vi "Boolean_To_String.vi"(4 "boolean":bool) -> (1 "string":string)   [LabVIEW 2016, in "PyLVi.lvlib" / "PyLVi.lvclass"]
uses:
  PyLVi.lvclass
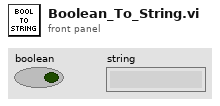
[diagram p1: front panel]
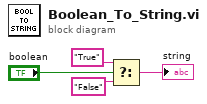
[diagram p0: block diagram]
diagram:
  n1 = Select(t="True", s="boolean", f="False") -> (s? t:f=→"string":string)
